vi "GetDataEvent_Service_2.vi"() -> ()   [LabVIEW 2017]
doc: "This is an example of how to read Data Sets from the InsightCM database. Using a similiar method you can read any waveform that has been stored and perform additional analysis on it or save it to a file format."
uses:
  <vilib>/addons/InsightCM/MessageBus/Base/controls/AssetNodeView.ctl
  <vilib>/addons/InsightCM/MessageBus/Base/controls/AssetState.ctl
  <vilib>/addons/InsightCM/MessageBus/Base/controls/Metric.ctl
  <vilib>/addons/InsightCM/MessageBus/Base/controls/KeyValuePair.ctl
  <vilib>/addons/InsightCM/MessageBus/Base/controls/AssetNodeReference.ctl
  <vilib>/addons/InsightCM/MessageBus/Base/controls/DataEvent.ctl
  <vilib>/addons/InsightCM/MessageBus/Base/controls/DataSetByteData.ctl
  <vilib>/addons/InsightCM/MessageBus/Base/controls/TrendPoint.ctl
  typedefs/Asset Info.ctl
  typedefs/Sensor Info.ctl
  typedefs/Metric Info.ctl
  typedefs/Q_Message.ctl
  <vilib>/addons/InsightCM/MessageBus/MessageService/IcmMessageService.lvclass
panel:
  out "LastTrendPoint":cluster{string, "Value":dbl}
  in  "String":string="This is an EXE to host a web service for InsightCM.\n\nhttp://127.0.0.1:8002/Query/GetLastEvent?Asset=<AssetName>\nOutput: Last event for the asset within X days, all channels (JSON)\n\nhttp://127.0.0.1:8002/Query/GetAssetList\nOutput: Asset ID, Sensor ID, and Metric ID (JSON)\n\nhttp://127.0.0.1:8002/Query/GetLastTrend?MetricID=<Metric ID of feature>\nOutput: Time and value of last trend point (JSON)"
  out "Trend":T1(graph)
  out "SIGMU Output":T2[](array[typedef])
  in  "Seconds from now":i64=3600
  out "error out":errorcluster
  out "Ready?":bool
  out "Parameter (debug)":string
  out "Command (debug)":string
  out "Output":T6(array[cluster])
  out "TrendPoints":T7[](array[typedef])
  out "DataSets":T8[](array[typedef])
  out "date/time":string
  out "Numeric":i32
  out "DataEvents":T9[](array[typedef])
  out "AssetNodeView":T10
  out "AssetNodes":T10[](array[typedef])
  # "1 hr = 3600, 1 day = 86400"
  # "This example shows how to query InsightCM data.\n\n1) Click Refresh to load assets.\n2) Select an asset.\n3) Select a data event and a sensor.\n\nNote: If the sensor does not have waveform data, the waveform graph will be empty."
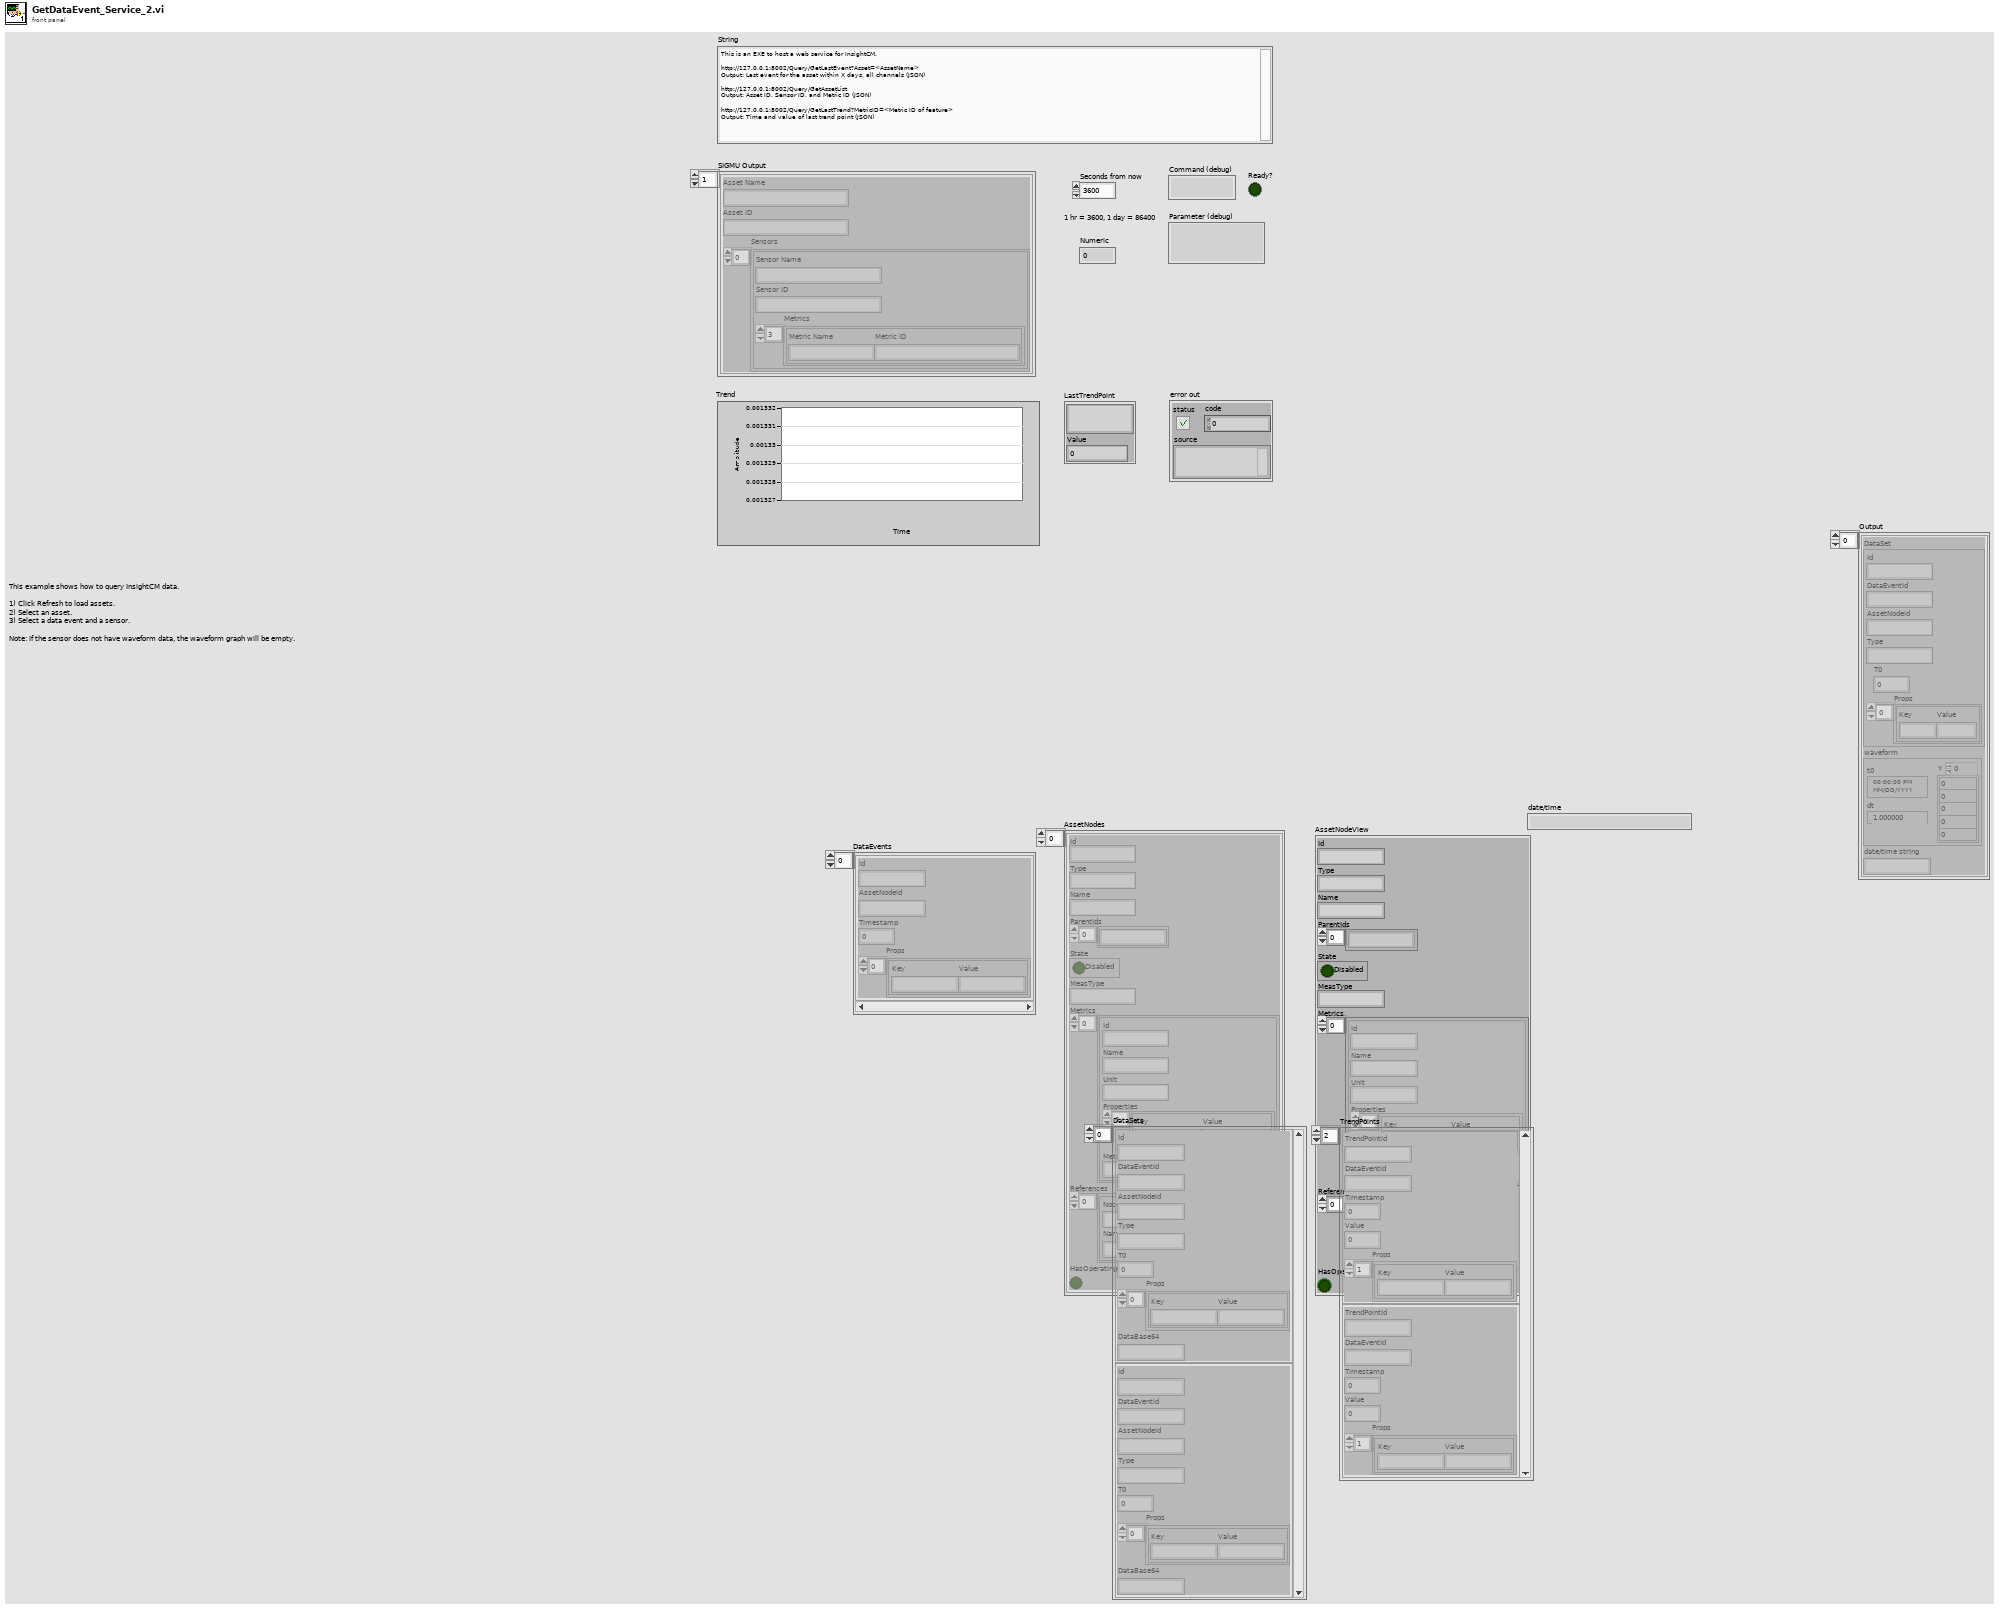
[diagram p1: front panel]
types:
  T1 = cluster{"Time Stamp out":timestamp, "Value":dbl}[]
  T2 = typedef "Asset Info.ctl" = cluster{"Asset Name":string, "Asset ID":string, "Sensors":T3[]}
  T3 = typedef "Sensor Info.ctl" = cluster{"Sensor Name":string, "Sensor ID":string, "Metrics":T4[]}
  T4 = typedef "Metric Info.ctl" = cluster{"Metric Name ":string, "Metric ID":string}
  T5 = typedef "KeyValuePair.ctl" = cluster{"Key":string, "Value":string}
  T6 = cluster{"DataSet":cluster{"Id":string, "DataEventId":string, "AssetNodeId":string, "Type":string, "T0":i64, "Props":T5[]}, "waveform":waveform(sgl), "date/time string":string}[]
  T7 = typedef "TrendPoint.ctl" = cluster{"TrendPointId":string, "DataEventId":string, "Timestamp":i64, "Value":dbl, "Props":T5[]}
  T8 = typedef "DataSetByteData.ctl" = cluster{"Id":string, "DataEventId":string, "AssetNodeId":string, "Type":string, "T0":i64, "Props":T5[], "DataBase64":string}
  T9 = typedef "DataEvent.ctl" = cluster{"Id":string, "AssetNodeId":string, "Timestamp":i64, "Props":T5[]}
  T10 = typedef "AssetNodeView.ctl" = cluster{"Id":string, "Type":string, "Name":string, "ParentIds":string[], "State":T11, "MeasType":string, "Metrics":T12[], "References":T13[], "HasOperatingStates":bool}
  T11 = typedef "AssetState.ctl" = cluster{"Disabled":bool}
  T12 = typedef "Metric.ctl" = cluster{"Id":string, "Name":string, "Unit":string, "Properties":T5[], "MetricDefinitionInstanceId":string}
  T13 = typedef "AssetNodeReference.ctl" = cluster{"NodeId":string, "Name":string}
  T14 = typedef "Q_Message.ctl" = cluster{"Command":string, "Parameters":variant}
  T15 = cluster{"Id":string, "DataEventId":string, "AssetNodeId":string, "Type":string, "T0":i64, "Props":T5[]}
  T16 = cluster{"DataSet":cluster{"Id":string, "DataEventId":string, "AssetNodeId":string, "Type":string, "T0":i64, "Props":T5[]}, "waveform":waveform(sgl), "date/time string":string}
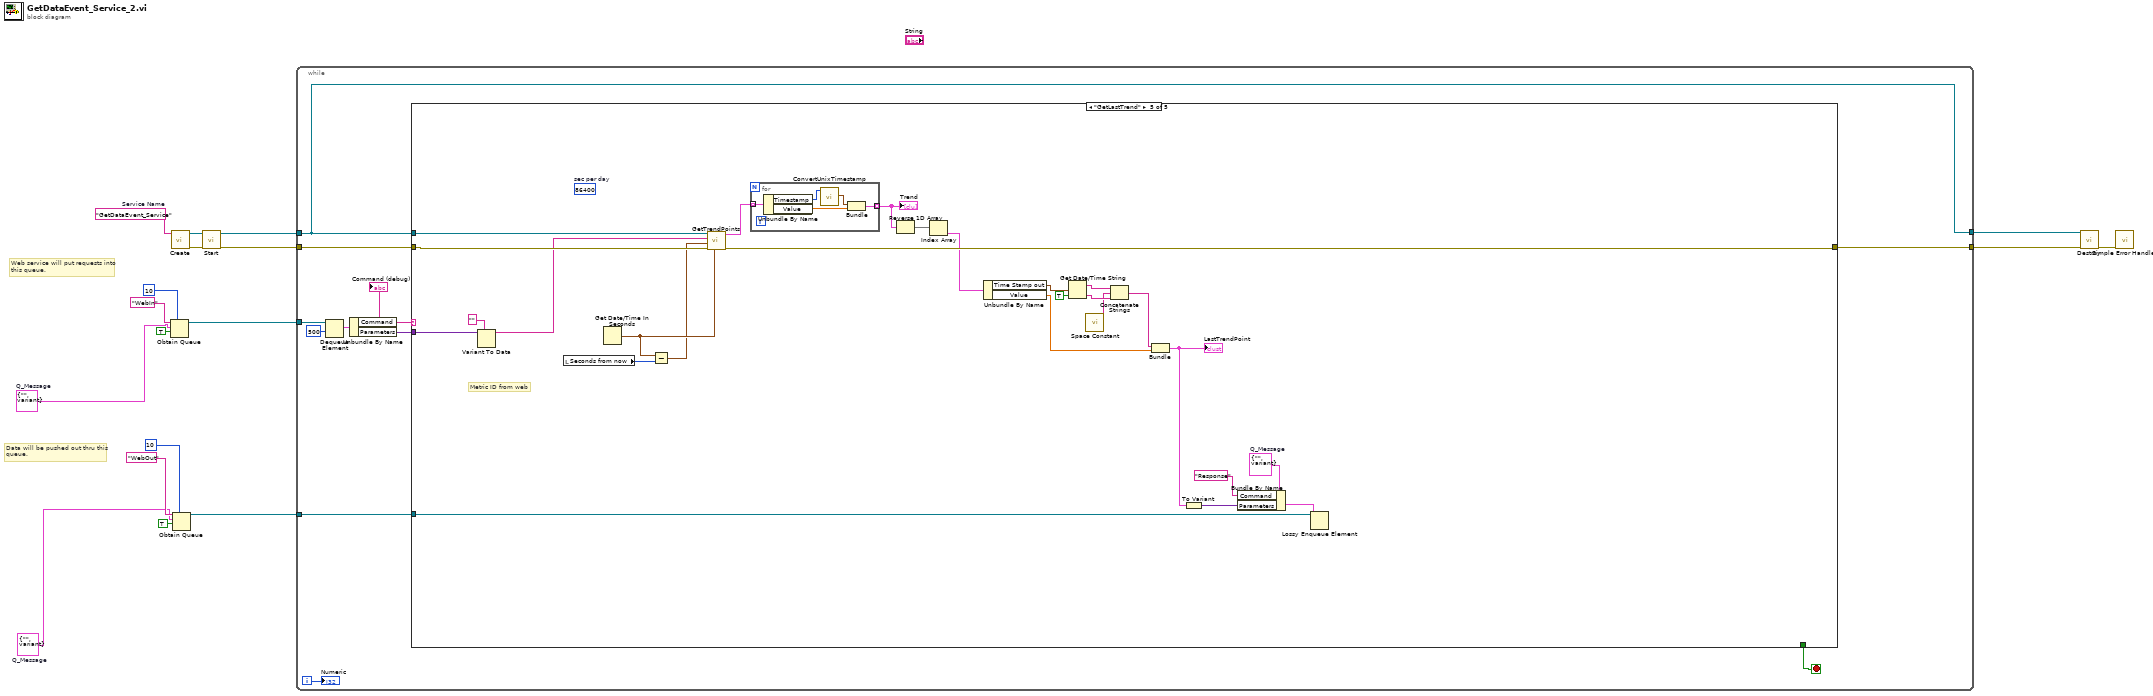
[diagram p0: block diagram]
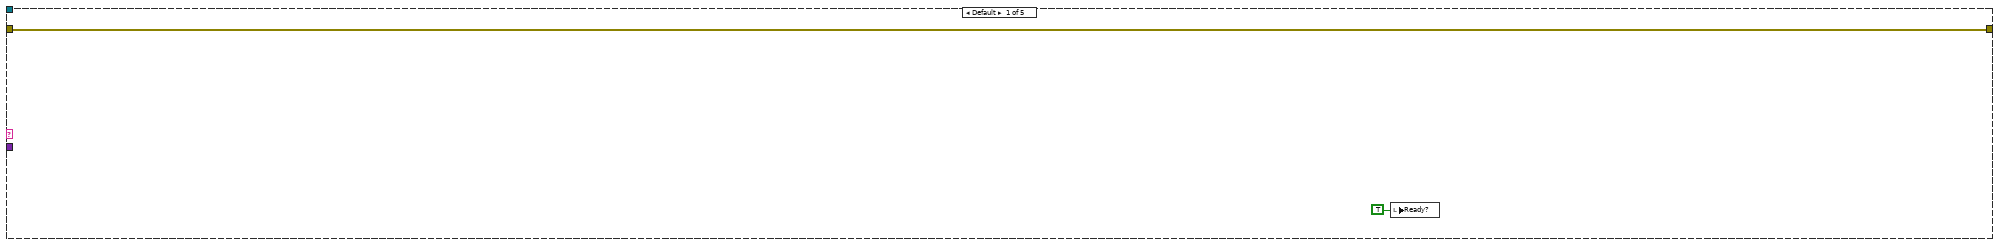
[diagram p2: hidden frame]
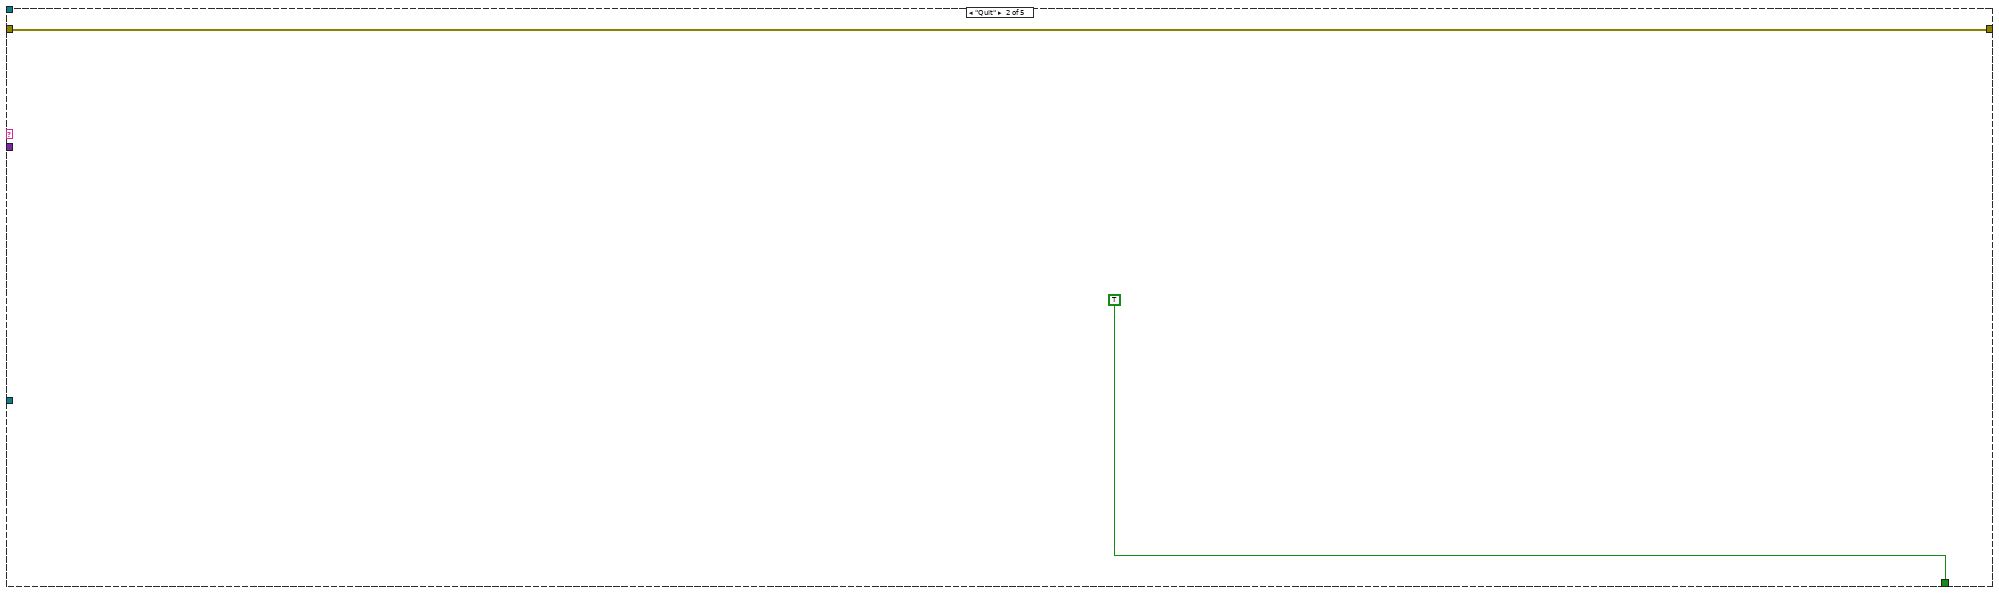
[diagram p3: hidden frame]
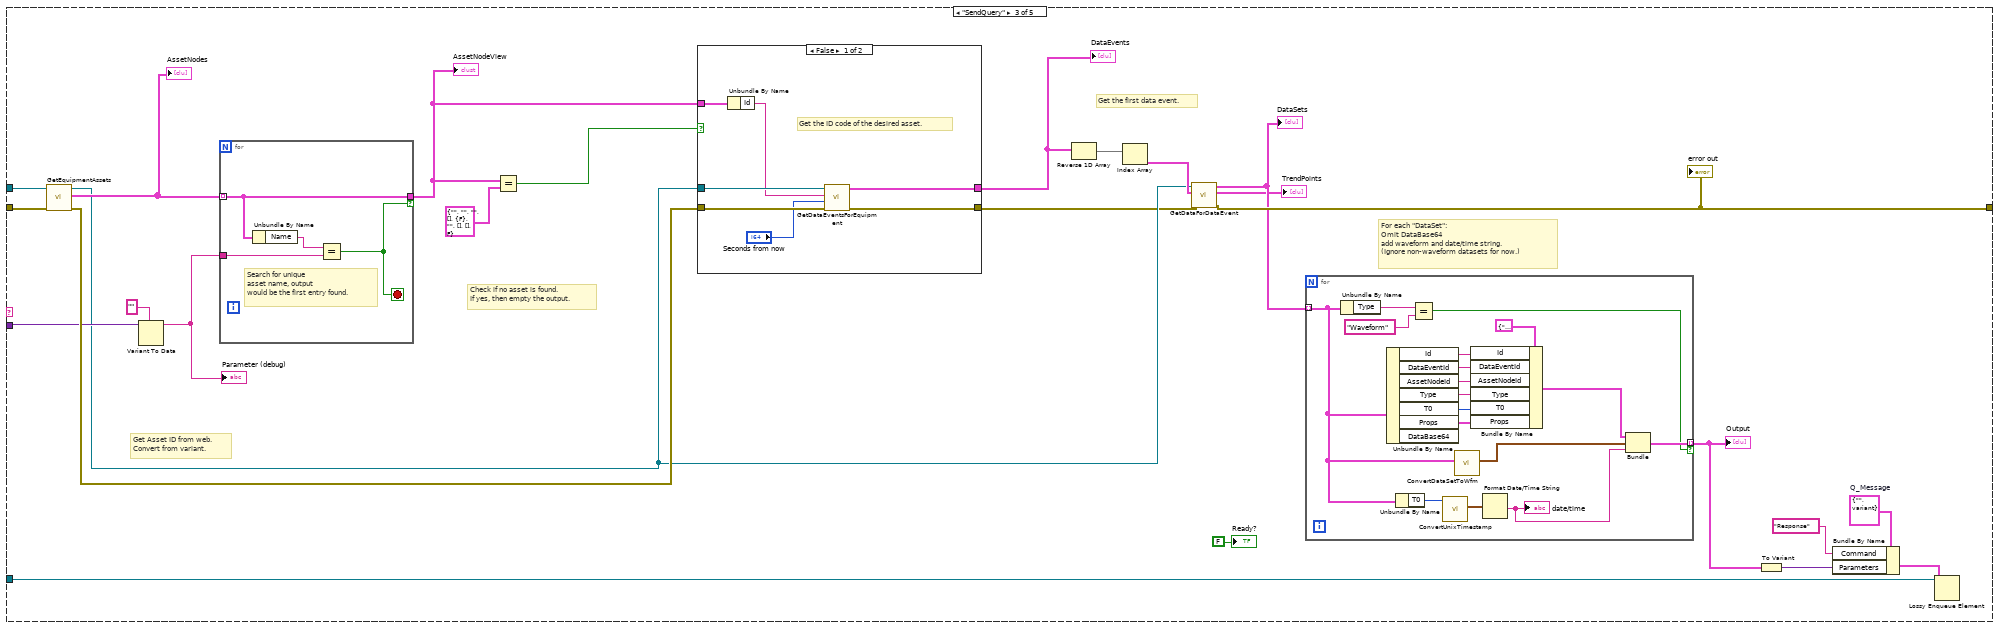
[diagram p4: hidden frame]
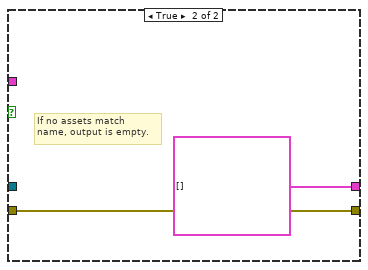
[diagram p5: hidden frame]
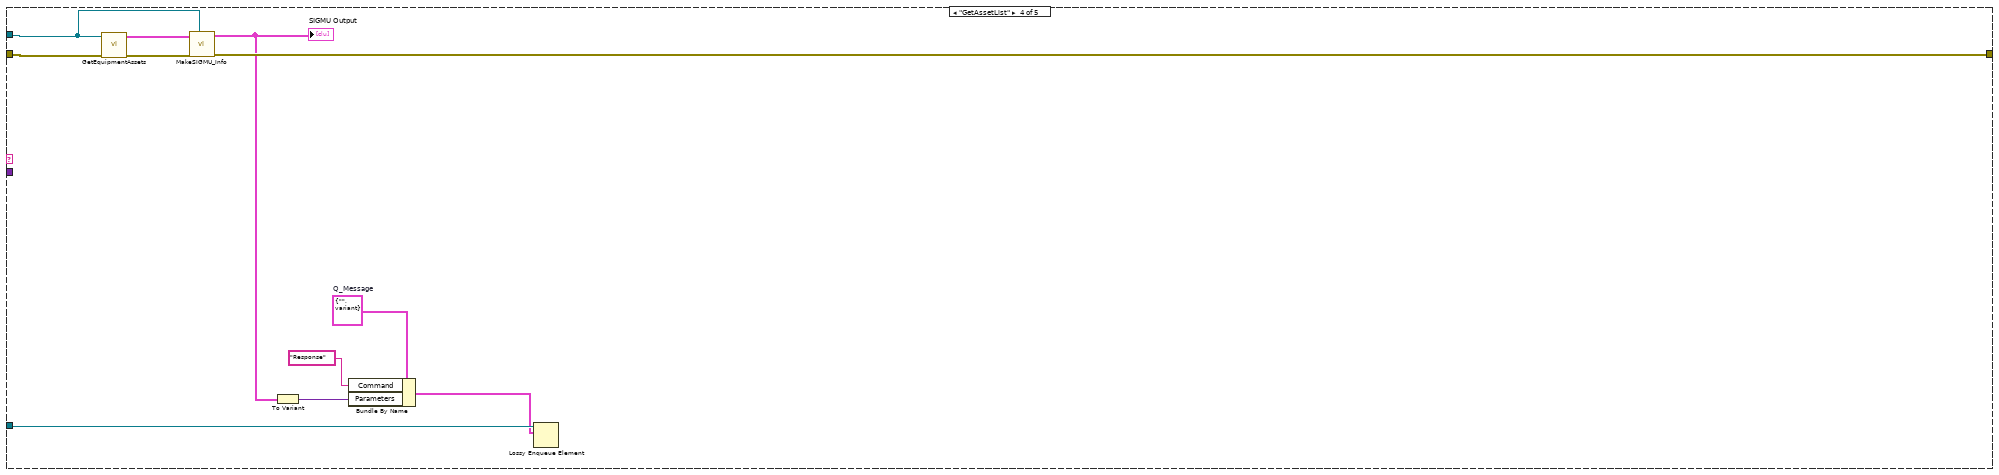
[diagram p6: hidden frame]
diagram:
  w1 = T14 {"Command"="", "Parameters"=variant}  # Q_Message
  w2 = T14 {"Command"="", "Parameters"=variant}  # Q_Message
  w18 = "GetDataEvent_Service"  # Service Name
  # "Data will be pushed out thru this\nqueue."
  # "Web service will put requests into\nthis queue."
  n1 = Obtain Queue(max queue size (-1, unlimited)=10, name (unnamed)="WebIn", element data type=w2, create if not found? (T)=TRUE) -> (queue out=w8:refnum<queue>)  [unwired: 1 in, 2 out]
  n2 = call <vilib>:"Create.vi"("service name"=w18) -> ("error out"=w13:errorcluster, "service out"=w14:refnum<class "IcmMessageService.lvclass">)  [unwired: 9 in]
  n3 = Obtain Queue(max queue size (-1, unlimited)=10, name (unnamed)="WebOut", element data type=w1, create if not found? (T)=TRUE) -> (queue out=w7:refnum<queue>)  [unwired: 1 in, 2 out]
  n4 = call <vilib>:"Start.vi"("error in (no error)"=w13, "service in"=w14) -> ("error out"=w11:errorcluster, "service out"=w12:refnum<class "IcmMessageService.lvclass">)  [unwired: 8 in]
  n5 = while {
    tunnel: w12 -> [w28]
    tunnel: w11 -> [w29]
    tunnel: [w28] -> w15
    tunnel: [w27] -> w16
    tunnel: w8 -> [w26]
    tunnel: w7 -> [w24]
    i -> [w19]
    stop <- w23 stop-if-true
    n6 = Dequeue Element(queue=w26, timeout in ms (-1)=500) -> (element=w22:T14)  [unwired: 1 in, 3 out]
    n7 = Unbundle By Name(w22) -> ("Command"=w21:string, "Parameters"=w20:variant)
    "Command (debug)" <- w21
    n8 = case shown="\"GetLastTrend\"" w21 {
      tunnel: w29 -> [w31 w33 w57 w98 w122]
      tunnel: w28 -> [_ _ w45 w96 w123]
      tunnel: [w31 w33 w43 w94 w115] -> w27
      tunnel: w24 -> [_ _ w36 w90 w108]
      tunnel: [_ TRUE _ _ _] -> w23
      tunnel: w20 -> [_ _ w51 _ w120]
      frame Default {
        n9 = local write "Ready?"(TRUE ("Ready?")) -> ()
      }
      frame "Quit" {
      }
      frame "SendQuery" {
        w34 = T14 {"Command"="", "Parameters"=variant}  # Q_Message
        # "For each \"DataSet\":\nOmit DataBase64\nadd waveform and date/time string.\n(Ignore non-waveform datasets for now.)"
        # "Get Asset ID from web.\nConvert from variant."
        # "Get the first data event."
        # "Check if no asset is found.\nIf yes, then empty the output."
        n10 = call "GetEquipmentAssets.vi"("error in (no error)"=w57, "service"=w45) -> ("error out"=w53:errorcluster, "AssetNodes"=w56:T10[])  [unwired: 8 in]
        "AssetNodes" <- w56
        n11 = Variant To Data(type="", Variant=w51) -> (data=w49:string)  [unwired: 1 in, 1 out]
        "Parameter (debug)" <- w49
        n12 = for {
          tunnel: w56 -> [w85] mode=indexing
          tunnel: w49 -> [w86]
          tunnel: [w85] -> w54 if=w84
          stop <- w84 stop-if-true
          # "Search for unique \nasset name, output\nwould be the first entry found."
          n13 = Unbundle By Name(w85) -> ("Name"=w87:string)
          n14 = Equal?(x=w87, y=w86) -> (x = y?=w84:bool)
        }
        "AssetNodeView" <- w54
        n15 = Equal?(x=w54, y=T10 {"Id"="", "Type"="", "Name"="", "ParentIds"=[], "State"={"Disabled"=FALSE}, "MeasType"="", "Metrics"=[], "References"=[], "HasOperatingStates"=FALSE} ("AssetNodeView 2")) -> (x = y?=w52:bool)
        n16 = case shown="False" w52 {
          tunnel: w54 -> [w79 _]
          tunnel: w45 -> [w81 _]
          tunnel: w53 -> [w80 w82]
          tunnel: [w78 T9[] [] ("DataEvents")] -> w48
          tunnel: [w77 w82] -> w44
          frame False {
            # "Get the ID code of the desired asset."
            n17 = Unbundle By Name(w79) -> ("Id"=w76:string)
            n18 = call "GetDataEventsForEquipment.vi"("error in (no error)"=w80, "sec per day"="Seconds from now", "equipment id"=w76, "service"=w81) -> ("error out"=w77:errorcluster, "DataEvents"=w78:T9[])  [unwired: 6 in]
          }
          frame True {
            # "If no assets match\nname, output is empty."
          }
        }
        "DataEvents" <- w48
        n19 = Reverse 1D Array(array=w48) -> (reversed array=w47:T9[])
        n20 = Index Array(array=w47) -> (element=w46:T9)  [unwired: 1 in]
        n21 = call "GetDataForDataEvent.vi"("error in (no error)"=w44, "DataEvent"=w46, "service"=w45) -> ("error out"=w43:errorcluster, "TrendPoints"=→"TrendPoints":T7[], "DataSets"=w42:T8[])  [unwired: 6 in]
        "DataSets" <- w42
        "error out" <- w43
        n22 = for {
          tunnel: w42 -> [w66] mode=indexing
          tunnel: [w68] -> w35 mode=indexing if=w67
          n23 = Unbundle By Name(w66) -> ("Type"=w74:string)
          n24 = Unbundle By Name(w66) -> ("Id"=w64:string, "DataEventId"=w60:string, "AssetNodeId"=w61:string, "Type"=w62:string, "T0"=w63:i64, "Props"=w59:T5[])  [unwired: 1 out]
          n25 = Unbundle By Name(w66) -> ("T0"=w72:i64)
          n26 = Equal?(x=w74, y="Waveform") -> (x = y?=w67:bool)
          n27 = call <vilib>:"ConvertUnixTimestamp.vi"("Timestamp in"=w72) -> ("Time Stamp out"=w71:timestamp)  [unwired: 10 in]
          n28 = call "ConvertDataSetToWfm.vi"("DataSet"=w66) -> ("waveform"=w70:waveform(sgl))  [unwired: 10 in]
          n29 = Bundle By Name(cluster=T15 {"Id"="", "DataEventId"="", "AssetNodeId"="", "Type"="", "T0"=0, "Props"=[]} ("DataSet"), "Id"=w64, "DataEventId"=w60, "AssetNodeId"=w61, "Type"=w62, "T0"=w63, "Props"=w59) -> (w58:T15)
          n30 = Format Date/Time String(seconds (now)=w71) -> (date/time string=w69:string)  [unwired: 2 in]
          "date/time" <- w69
          n31 = Bundle("DataSet"=w58, "waveform"=w70, "date/time string"=w69) -> (w68:T16)  [unwired: 1 in]
        }
        "Output" <- w35
        n32 = To Variant(anything=w35) -> (Variant=w38:variant)
        n33 = Bundle By Name(cluster=w34, "Command"="Response", "Parameters"=w38) -> (w37:T14)
        n34 = Lossy Enqueue Element(queue=w36, element=w37) -> ()  [unwired: 1 in, 4 out]
        "Ready?" <- FALSE ("Ready?")
      }
      frame "GetAssetList" {
        w88 = T14 {"Command"="", "Parameters"=variant}  # Q_Message
        n35 = call "GetEquipmentAssets.vi"("error in (no error)"=w98, "service"=w96) -> ("error out"=w95:errorcluster, "AssetNodes"=w97:T10[])  [unwired: 8 in]
        n36 = call "MakeSIGMU_Info.vi"("ICM Service in"=w96, "error in (no error)"=w95, "AssetNodes In"=w97) -> ("error out"=w94:errorcluster, "SIGMU Output"=w93:T2[])  [unwired: 7 in]
        "SIGMU Output" <- w93
        n37 = To Variant(anything=w93) -> (Variant=w91:variant)
        n38 = Bundle By Name(cluster=w88, "Command"="Response", "Parameters"=w91) -> (w89:T14)
        n39 = Lossy Enqueue Element(queue=w90, element=w89) -> ()  [unwired: 1 in, 4 out]
      }
      frame "GetLastTrend" {
        w109 = T14 {"Command"="", "Parameters"=variant}  # Q_Message
        (unwired) 86400  # sec per day
        # "Metric ID from web"
        n40 = Variant To Data(type="", Variant=w120) -> (data=w119:string)  [unwired: 1 in, 1 out]
        n41 = local read "Seconds from now"() -> (w117:i64)
        n42 = Get Date/Time In Seconds() -> (seconds since 1Jan1904=w118:timestamp)
        n43 = Subtract(x=w118, y=w117) -> (x-y=w116:timestamp)
        n44 = call "GetTrendPoints.vi"("End Time"=w118, "error in (no error)"=w122, "Start Time"=w116, "trend id"=w119, "service"=w123) -> ("error out"=w115:errorcluster, "TrendPoints"=w124:T7[])  [unwired: 5 in]
        n45 = for {
          tunnel: w124 -> [w129] mode=indexing
          tunnel: [w128] -> w113 mode=indexing
          n46 = Unbundle By Name(w129) -> ("Timestamp"=w126:i64, "Value"=w127:dbl)
          n47 = call <vilib>:"ConvertUnixTimestamp.vi"("Timestamp in"=w126) -> ("Time Stamp out"=w125:timestamp)  [unwired: 10 in]
          n48 = Bundle("Time Stamp out"=w125, "Value"=w127) -> (w128:cluster{"Time Stamp out":timestamp, "Value":dbl})  [unwired: 1 in]
        }
        "Trend" <- w113
        n49 = Reverse 1D Array(array=w113) -> (reversed array=w114:T1)
        n50 = Index Array(array=w114) -> (element=w100:cluster{"Time Stamp out":timestamp, "Value":dbl})  [unwired: 1 in]
        n51 = Unbundle By Name(w100) -> ("Time Stamp out"=w107:timestamp, "Value"=w101:dbl)
        n52 = Get Date/Time String(seconds (now)=w107, want seconds? (F)=TRUE) -> (date string=w105:string, time string=w104:string)  [unwired: 1 in]
        n53 = call <vilib>:"Space Constant.vi"() -> ("String"=w103:string)
        n54 = Concatenate Strings(w105, w103, w104) -> (w102:string)
        n55 = Bundle(w102, "Value"=w101) -> (w99:cluster{string, "Value":dbl})  [unwired: 1 in]
        "LastTrendPoint" <- w99
        n56 = To Variant(anything=w99) -> (Variant=w111:variant)
        n57 = Bundle By Name(cluster=w109, "Command"="Response", "Parameters"=w111) -> (w110:T14)
        n58 = Lossy Enqueue Element(queue=w108, element=w110) -> ()  [unwired: 1 in, 4 out]
      }
    }
    "Numeric" <- w19
  }
  n59 = call <vilib>:"Destroy.vi"("error in (no error)"=w16, "service in"=w15) -> ("error out"=w17:errorcluster)  [unwired: 9 in]
  n60 = call <vilib>:"Simple Error Handler.vi"("error in (no error)"=w17) -> ()  [unwired: 4 in, 5 out]
